vi "INIT.vi"(8 "error in (no error)":errorcluster, 11 "UI Actor in":refnum<class "UI Actor.lvclass">) -> (0 "error out":errorcluster, 3 "UI Actor out":refnum<class "UI Actor.lvclass">)   [LabVIEW 2019, in "UI Actor.lvlib" / "UI Actor.lvclass"]
uses:
  UI Actor.lvclass
  C:/Program Files (x86)/National Instruments/LabVIEW 2019/vi.lib/ActorFramework/Actor/Actor.lvclass
  UI Actor.lvclass/UI Actor.ctl
  MXN ACTOR/MXN ACTOR.lvclass
  MXN ACTOR/MXN ACTOR.lvclass/MXN ACTOR.ctl
  USD ACTOR/USD ACTOR.lvclass
  USD ACTOR/USD ACTOR.lvclass/USD ACTOR.ctl
  Soda Actor/Soda Actor.lvclass
  Soda Actor/Soda Actor.lvclass/Soda Actor.ctl
  coffee Actor/coffee Actor.lvclass
  coffee Actor/coffee Actor.lvclass/coffee Actor.ctl
  Read Coins.vi
  Read Sub panel coin.vi
  Read Productos.vi
  Read Sub panel Prod.vi
  <vilib>/ActorFramework/Actor/Actor.lvclass
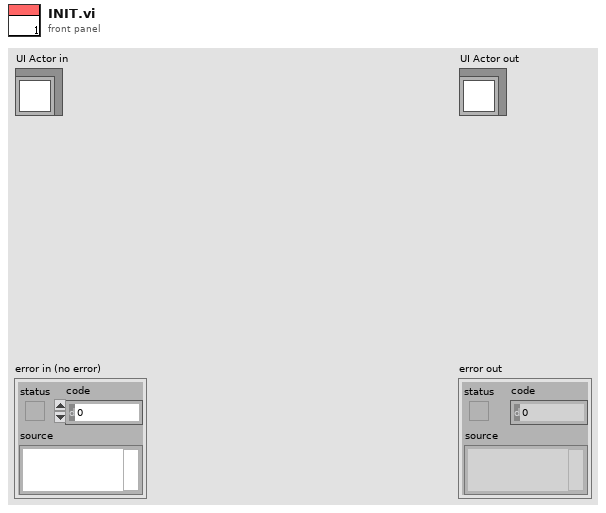
[diagram p1: front panel]
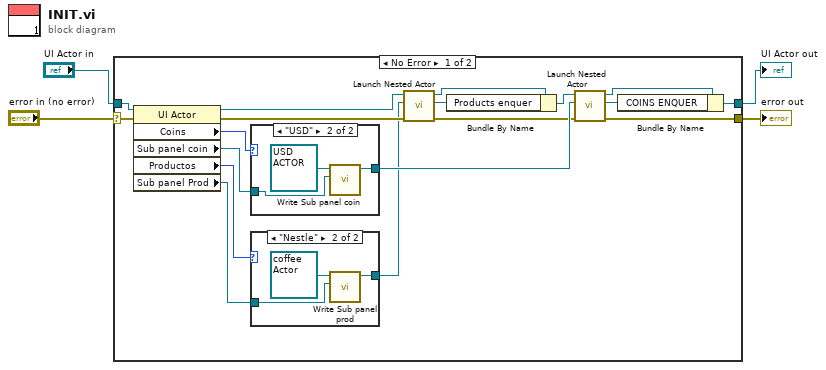
[diagram p0: block diagram]
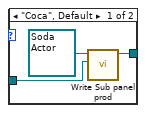
[diagram p2: hidden frame]
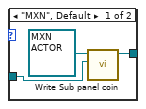
[diagram p3: hidden frame]
diagram:
  n1 = case shown="No Error" "error in (no error)" {
    selector: "error in (no error)" -> [w21 w36]
    tunnel: [w19 w36] -> w3
    tunnel: [w17 w35] -> w1
    tunnel: "UI Actor in" -> [w22 w35]
    frame No Error {
      n2 = property class="UI Actor"(reference=w22, error in=w21) -> (reference out=w9:refnum<class "UI Actor.lvclass">, error out=w11:errorcluster, "Coins"=w20:enum16{"MXN", "USD", ""}, "Sub panel coin"=w14:refnum<vi>, "Productos"=w13:enum16{"Coca", "Nestle"}, "Sub panel Prod"=w12:refnum<vi>)
      n3 = case shown="\"USD\"" w20 {
        tunnel: [w30 w32] -> w18
        tunnel: w14 -> [w29 w33]
        frame "MXN", Default {
          n4 = call "Write Sub panel coin.vi"("Sub panel coin"=w29, "MXN ACTOR in"=refnum<class "MXN ACTOR.lvclass"> refnum ("MXN ACTOR.lvlib:MXN ACTOR.lvclass")) -> ("MXN ACTOR out"=w30:refnum<class "MXN ACTOR.lvclass">)  [unwired: 8 in, 1 out]
        }
        frame "USD" {
          n5 = call "Write Sub panel coin.vi"("Sub panel coin"=w33, "USD ACTOR in"=refnum<class "USD ACTOR.lvclass"> refnum ("USD ACTOR.lvlib:USD ACTOR.lvclass")) -> ("USD ACTOR out"=w32:refnum<class "USD ACTOR.lvclass">)  [unwired: 8 in, 1 out]
        }
      }
      n6 = case shown="\"Nestle\"" w13 {
        tunnel: w12 -> [w24 w27]
        tunnel: [w23 w26] -> w8
        frame "Coca", Default {
          n7 = call "Write Sub panel prod.vi"("Sub panel prod"=w24, "Soda Actor in"=refnum<class "Soda Actor.lvclass"> refnum ("Soda Actor.lvlib:Soda Actor.lvclass")) -> ("Soda Actor out"=w23:refnum<class "Soda Actor.lvclass">)  [unwired: 8 in, 1 out]
        }
        frame "Nestle" {
          n8 = call "Write Sub panel prod.vi"("Sub panel prod"=w27, "coffee Actor in"=refnum<class "coffee Actor.lvclass"> refnum ("coffee Actor.lvlib:coffee Actor.lvclass")) -> ("coffee Actor out"=w26:refnum<class "coffee Actor.lvclass">)  [unwired: 8 in, 1 out]
        }
      }
      n9 = call <vilib>:"Launch Nested Actor.vi"("error in (no error)"=w11, "Nested Actor"=w8, "Caller Actor in"=w9) -> ("error out"=w10:errorcluster, "Nested Actor's Enqueuer"=w5:refnum<class "Message Enqueuer.lvclass">, "Caller Actor out"=w7:refnum<class "UI Actor.lvclass">)  [unwired: 6 in]
      n10 = Bundle By Name(cluster=w7, "Products enquer"=w5) -> (w6:refnum<class "UI Actor.lvclass">)
      n11 = call <vilib>:"Launch Nested Actor.vi"("error in (no error)"=w10, "Nested Actor"=w18, "Caller Actor in"=w6) -> ("error out"=w19:errorcluster, "Nested Actor's Enqueuer"=w15:refnum<class "Message Enqueuer.lvclass">, "Caller Actor out"=w16:refnum<class "UI Actor.lvclass">)  [unwired: 6 in]
      n12 = Bundle By Name(cluster=w16, "COINS ENQUER"=w15) -> (w17:refnum<class "UI Actor.lvclass">)
    }
    frame Error {
    }
  }
  "error out" <- w3
  "UI Actor out" <- w1
